vi "drivable or random paths (subsumption).vi"(1 "driveable drive vectors":i8[](array[numeric])=[0, 0, 0, 0, 0, 0, 0, 0, 0], 2 "possible drive vectors":i8[](array[numeric])=[0, 0, 0, 0, 0, 0, 0, 0, 0]) -> (6 "choosen drive vectors":i8[](array[numeric]))   [LabVIEW 2009]
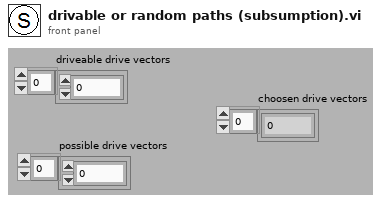
[diagram p1: front panel]
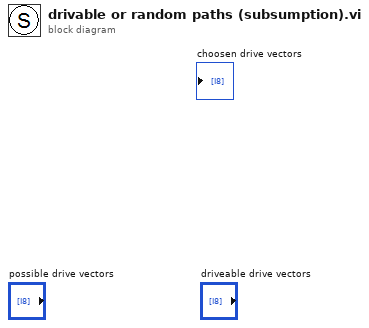
[diagram p0: block diagram]
diagram:
